vi "Change_RunInfo.vi"(2 "error in (no error)":errorcluster, 3 "Run Data SubPanel in":T1) -> (0 "error out":errorcluster, 1 "Run Data SubPanel out":T1)   [LabVIEW 2019]
uses:
  Controls/DataBlockControl.ctl
panel:
  in  "Apply Changes":bool
  out "Current Run Data":T1
  in  "Exit SubVI":bool
  in  "Run Data Input":T1
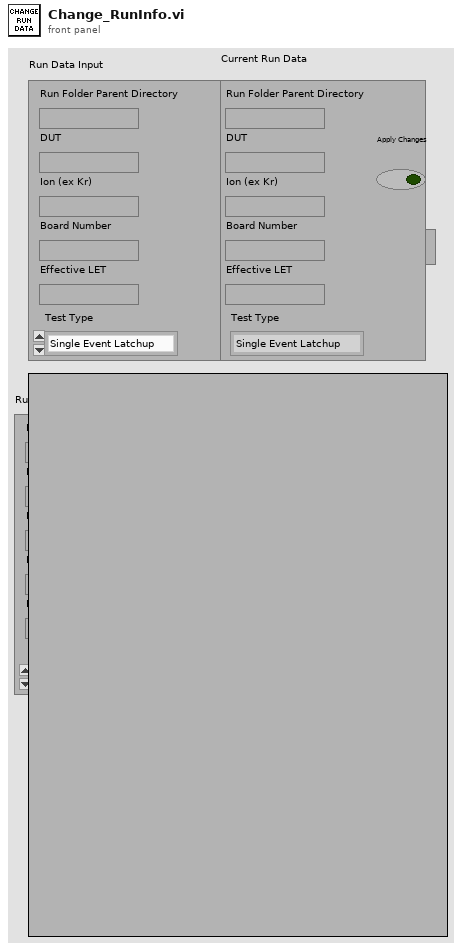
[diagram p1: front panel]
types:
  T1 = typedef "DataBlockControl.ctl" = cluster{"Run Folder Parent Directory":path, "DUT":string, "Ion (ex Kr)":string, "Board Number":string, "Effective LET":string, "Test Type":enum16{"Single Event Latchup", "Single Event Transient", "Single Event Upset"}}
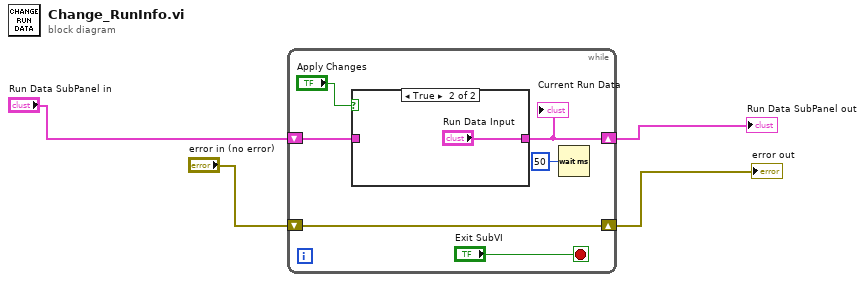
[diagram p0: block diagram]
diagram:
  n1 = while {
    shift-right: [w8] -> w4
    shift-left: "Run Data SubPanel in" -> [w5]
    shift-right: [w7] -> w2
    shift-left: "error in (no error)" -> [w7]
    stop <- "Exit SubVI" stop-if-true
    n2 = case shown="True" "Apply Changes" {
      tunnel: [w11 "Run Data Input"] -> w8
      tunnel: w5 -> [w11 _]
      frame False {
      }
      frame True {
      }
    }
    "Current Run Data" <- w8
    n3 = Wait (ms)(milliseconds to wait=u32 50) -> ()  [unwired: 1 out]
  }
  "Run Data SubPanel out" <- w4
  "error out" <- w2
